vi "Check Status.vi"(7 "Source (\"\")":string, 8 "Error In":errorcluster, 10 "Status":i32, 11 "libssh2lv Shared Library In":path=path "") -> (0 "Error Out":errorcluster, 3 "libssh2lv Shared Library Out":path)   [LabVIEW 2021, in "Field_RnD_Services_LIBSSH2_Toolkit.lvlib"]
doc: "Determines the result of the function call from the libssh2lv shared library and converts failures to an error."
uses:
  Field_RnD_Services_LIBSSH2_Toolkit.lvlib
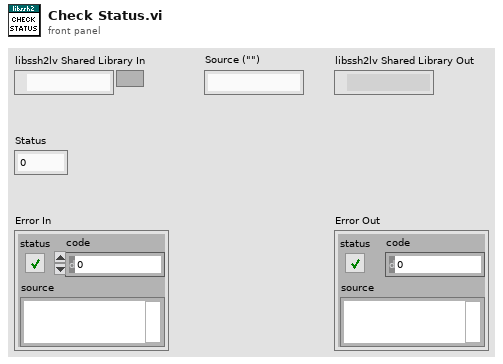
[diagram p1: front panel]
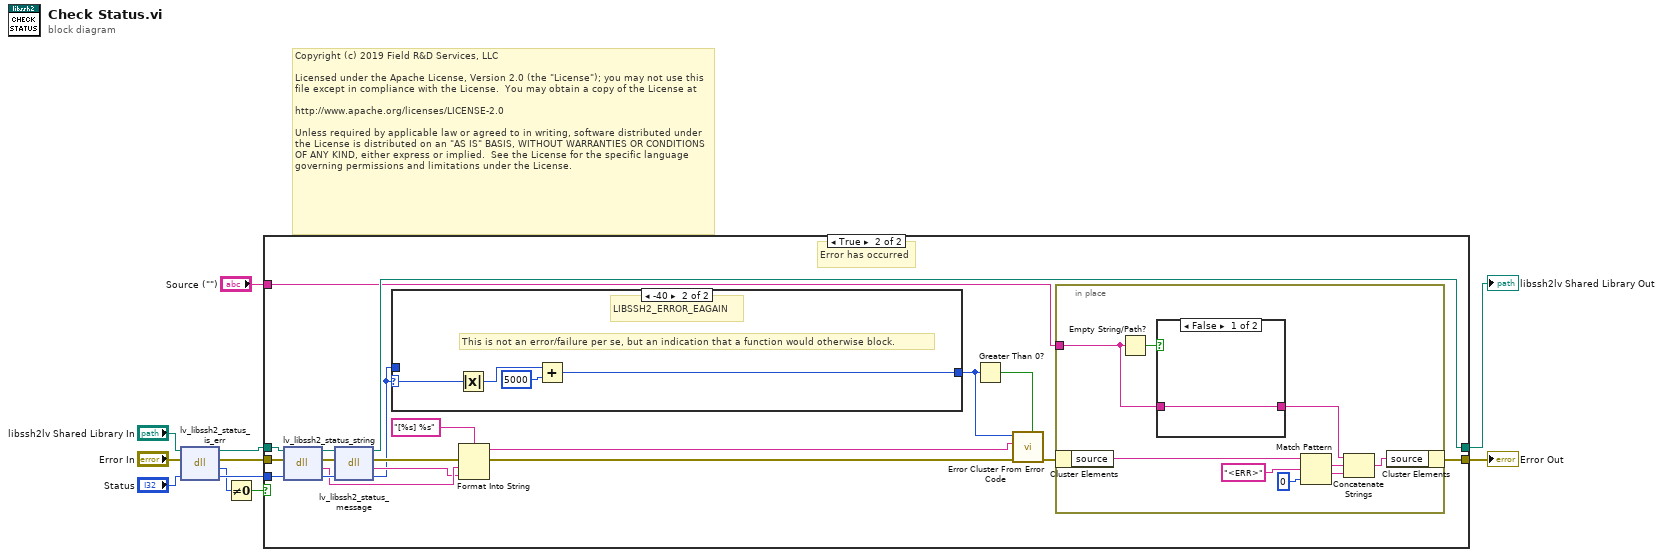
[diagram p0: block diagram]
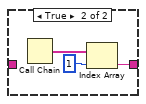
[diagram p3: hidden frame]
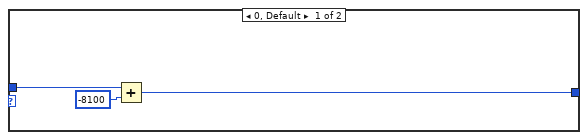
[diagram p4: hidden frame]
diagram:
  # "Copyright (c) 2019 Field R&D Services, LLC\n\nLicensed under the Apache License, Version 2.0 (the \"License\"); you may not use this file except in compliance with the License.  You may obtain a copy of the License at\n\nhttp://www.apache.org/licenses/LICENSE-2.0\n\nUnless required by applicable law or agreed to in writing, software distributed under the License is distributed on an \"AS IS\" BASIS, WITHOUT WARRANTIES OR CONDITIONS OF ANY KIND, either express or implied.  See the License for the specific language governing permissions and limitations under the License."
  n1 = dll-call lib="libssh2lv.*" fn="lv_libssh2_status_is_err"(path in="libssh2lv Shared Library In", error in="Error In", "status"="Status") -> (path out=w10:path, error out=w8:errorcluster, "bool"=w3:i32, "status"=w6:i32)  [unwired: 1 in]
  n2 = Not Equal To 0?(x=w3) -> (x != 0?=w2:bool)
  n3 = case shown="True" w2 {
    tunnel: w10 -> [w13 w29]
    tunnel: w8 -> [w12 w28]
    tunnel: w6 -> [_ w27]
    tunnel: [w13 w26] -> w5
    tunnel: [w12 w15] -> w4
    tunnel: "Source (\"\")" -> [_ w14]
    frame False {
      # "No error"
    }
    frame True {
      # "Error has occurred"
      n4 = dll-call lib="libssh2lv.*" fn="lv_libssh2_status_string"(path in=w29, error in=w28, "status"=w27) -> (path out=w30:path, error out=w31:errorcluster, "string"=w21:string, "status"=w32:i32)  [unwired: 1 in]
      n5 = dll-call lib="libssh2lv.*" fn="lv_libssh2_status_message"(path in=w30, error in=w31, "status"=w32) -> (path out=w26:path, error out=w24:errorcluster, "message"=w20:string, "status"=w19:i32)  [unwired: 1 in]
      n6 = case shown="-40" w19 {
        selector: w19 -> [_ w52]
        tunnel: w19 -> [w47 _]
        tunnel: [w46 w49] -> w18
        frame 0, Default {
          n7 = Add(x=w47, y=-8100) -> (x+y=w46:i32)
        }
        frame -40 {
          # "This is not an error/failure per se, but an indication that a function would otherwise block."
          # "LIBSSH2_ERROR_EAGAIN"
          n8 = Absolute Value(x=w52) -> (abs(x)=w51:i32)
          n9 = Add(x=w51, y=5000) -> (x+y=w49:i32)
        }
      }
      n10 = Format Into String(format string="[%s] %s", error in=w24, w21, w20) -> (resulting string=w22:string, error out=w23:errorcluster)  [unwired: 1 in]
      n11 = Greater Than 0?(x=w18) -> (x > 0?=w17:bool)
      n12 = call <vilib>:"Error Cluster From Error Code.vi"("is warning? (False)"=w17, "error in (no error)"=w23, "error message (\"\")"=w22, "error code (0)"=w18) -> ("error out"=w16:errorcluster)  [unwired: 5 in]
      n13 = in-place {
        in-place-border: w14 -> [w33]
        n14 = in-place-cluster #1(w16) -> ("source"=w39:string)
        n15 = Empty String/Path?(string/path=w33) -> (empty?=w35:bool)
        n16 = case shown="False" w35 {
          tunnel: [w42 w43] -> w34
          tunnel: w33 -> [w42 _]
          frame False {
          }
          frame True {
            n17 = Call Chain() -> (call chain=w45:string[])
            n18 = Index Array(array=w45, index=1) -> (element=w43:string)
          }
        }
        n19 = Match Pattern(string=w39, regular expression="<ERR>", offset (0)=0) -> (match substring=w38:string, after substring=w37:string)  [unwired: 2 out]
        n20 = Concatenate Strings(w34, w38, w37) -> (w36:string)
        n21 = in-place-cluster #1("source"=w36) -> (w15:errorcluster)
      }
    }
  }
  "libssh2lv Shared Library Out" <- w5
  "Error Out" <- w4
